vi "edit io channel.vi"(6 "refresh UI":T2, 8 "error in":errorcluster, 9 "PID Loop Element":T1={"Loop ID"="", "Tags"={"Setpoint"="", "Process Variable"="", "Output"=""}, "Gains"={"P"=1.0, "I"=0.01, "D"=0.0}, "Range"={"High"=100.0, "Low"=-100.0}}, 10 "engine configuration in":refnum<class "engine configuration.lvclass">, 11 "tag bus configurable plugin module configuration in":refnum<class "PID Module configuration.lvclass">) -> (0 "error out":errorcluster, 1 "change?":bool, 2 "engine configuration":refnum<class "engine configuration.lvclass">, 3 "tag bus configurable plugin module configuration out":refnum<class "PID Module configuration.lvclass">)   [LabVIEW 2014, in "PID Module editor node.lvclass"]
uses:
  PID Module editor node.lvclass
  <vilib>/NI/Configuration Framework/Node/RefreshUIEvent.ctl
  <vilib>/NI/Module Execution Interface/Engine Configuration/engine configuration.lvclass
  module/configuration/PID Module configuration.lvclass
  PID array element.ctl
  <vilib>/NI/Configuration Framework/Node/NISE_CEF_Node.lvclass
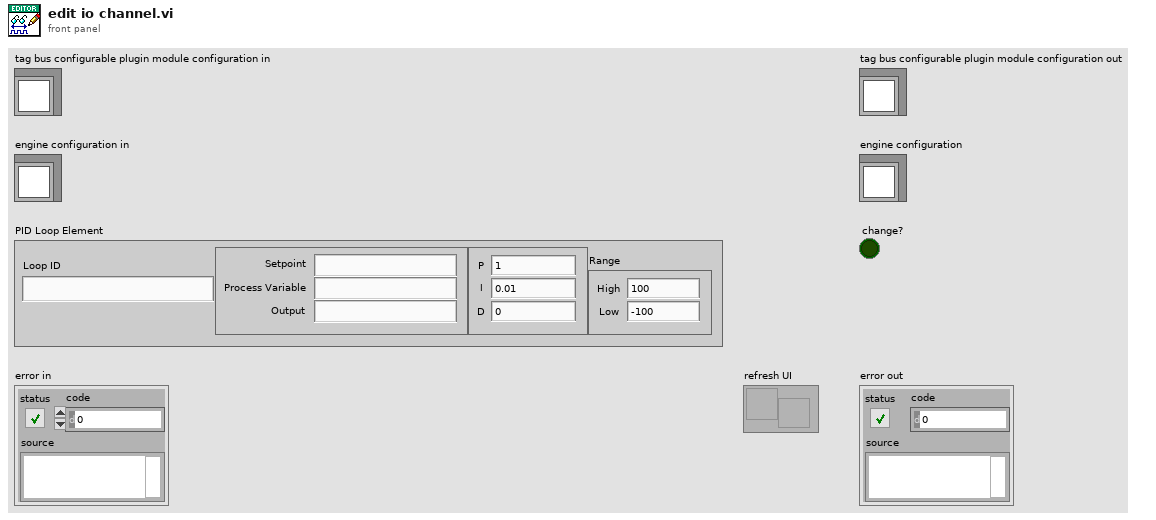
[diagram p1: front panel]
types:
  T1 = typedef "PID Module editor node.lvclass/PID array element.ctl" = cluster{"Loop ID":string, "Tags":cluster{"Setpoint":string, "Process Variable":string, "Output":string}, "Gains":cluster{"P":dbl, "I":dbl, "D":dbl}, "Range":cluster{"High":dbl, "Low":dbl}}
  T2 = typedef "NISE_CEF_Node.lvclass/RefreshUIEvent.ctl" = refnum<user-event>
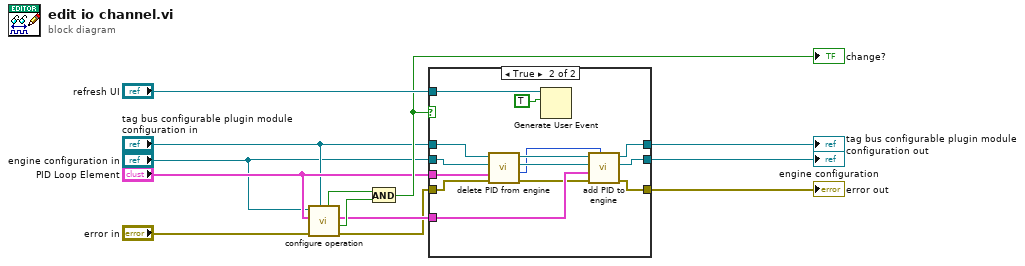
[diagram p0: block diagram]
diagram:
  n1 = call "configure operation.vi"("tag bus configurable plugin module configuration"="tag bus configurable plugin module configuration in", "error in"="error in", "line item in"="PID Loop Element", "engine configuration"="engine configuration in") -> ("error out"=w6:errorcluster, "success"=w10:bool, "PID Loop out"=w7:T1, "changed"=w9:bool)  [unwired: 4 in]
  n2 = And(x=w9, y=w10) -> (x .and. y?=w11:bool)
  "change?" <- w11
  n3 = case shown="True" w11 {
    tunnel: [w16 w21] -> w5
    tunnel: [w14 w22] -> w3
    tunnel: "engine configuration in" -> [w14 w25]
    tunnel: w6 -> [w16 w24]
    tunnel: w7 -> [_ w28]
    tunnel: "PID Loop Element" -> [_ w27]
    tunnel: "tag bus configurable plugin module configuration in" -> [w15 w26]
    tunnel: [w15 w23] -> w12
    tunnel: "refresh UI" -> [_ w30]
    frame False {
    }
    frame True {
      n4 = call "delete PID from engine.vi"("error in (no error)"=w24, "PID Loop in"=w27, "engine configuration in"=w25, "Tagbus PID Module configuration in"=w26) -> ("error out"=w20:errorcluster, "index"=w17:i32, "engine configuration out"=w19:refnum<class "engine configuration.lvclass">, "Tagbus PID Module configuration out"=w18:refnum<class "PID Module configuration.lvclass">)  [unwired: 4 in]
      n5 = Generate User Event(user event=w30, event data cluster=TRUE ("event data")) -> ()  [unwired: 2 in, 2 out]
      n6 = call "add PID to engine.vi"("index"=w17, "error in (no error)"=w20, "PID element in"=w28, "engine configuration"=w19, "Tagbus PID Module configuration in"=w18) -> ("error out"=w21:errorcluster, "engine configuration out"=w22:refnum<class "engine configuration.lvclass">, "Tagbus PID Module configuration out"=w23:refnum<class "PID Module configuration.lvclass">)  [unwired: 4 in]
    }
  }
  "engine configuration" <- w3
  "tag bus configurable plugin module configuration out" <- w12
  "error out" <- w5
